vi "_074.vi"() -> ()   [LabVIEW 2024]
panel:
  out "5":i32
  out "x/y":dbl
  in  "x":dbl
  in  "y":dbl
  out "4":i32
  out "3":i32
  out "2":i32
  out "1":i32
  out "o/p":i32
  # "Fundamentals :"
  # "3~>After running this VI,what is the value displayed in the o/p ?"
  # "Nrml Approach :"
  # "Dfrnt Approach :"
  # "( Work flow )"
  # "I learned in this question in To get the index val (in 1-D array only positive indexes) if the i/p is positive, then the o/p is the i/p's index val.\nThe default of the negative index & the undefined index is zero"
  # "I learned one more in this question What is NaN , The NaN is ( Not a Number ) works in this case ZERO Divided by ZERO. The infinity called as NaN in LabVIEW ."
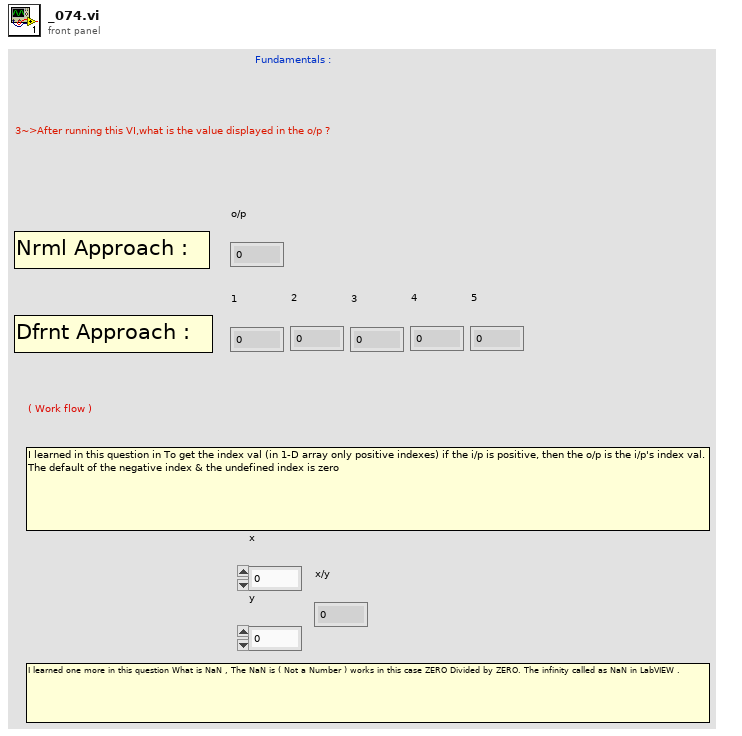
[diagram p1: front panel]
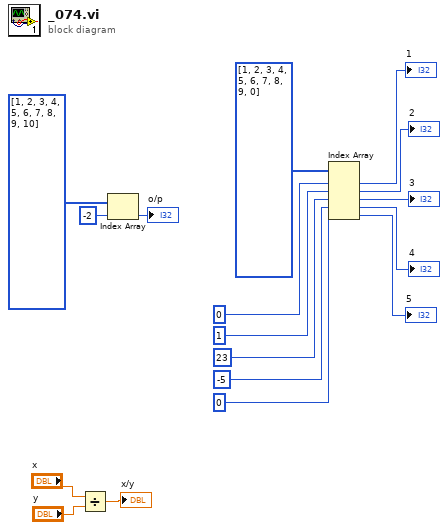
[diagram p0: block diagram]
diagram:
  n1 = Divide(x="x", y="y") -> (x/y=→"x/y":dbl)
  n2 = Index Array "Index Array"(array=i32[] [1, 2, 3, 4, 5, 6, 7, 8, 9, 10], index=-2) -> (element=→"o/p":i32)
  n3 = Index Array "Index Array"(array=i32[] [1, 2, 3, 4, 5, 6, 7, 8, 9, 0], index #1=0, index #2=1 ("index"), index #3=23 ("index"), index #4=-5 ("index"), index #5=0 ("index")) -> (element #1=→"1":i32, element #2=→"2":i32, element #3=→"3":i32, element #4=→"4":i32, element #5=→"5":i32)
